vi "Apply VIignore File.vi"(8 "error in":errorcluster, 10 ".VIignore file":path, 11 "VI paths in":path[](array[path])) -> (0 "error out":errorcluster, 2 "Filtered files":string[](array[string]), 3 "VI paths filtered":path[](array[path]))   [LabVIEW 2020, in "CICD.lvlib"]
doc: "Takes in an array of paths and filters them based on filenames in .VIignore file."
uses:
  CICD.lvlib
  65742ef6-5497-4067-8f50-dc0572609d26.vi
  65742ef6-5497-4067-8f50-dc0572609d26.vi/7c7783df-fd5a-49d9-9b7a-63cc9fb0e4e5.vi
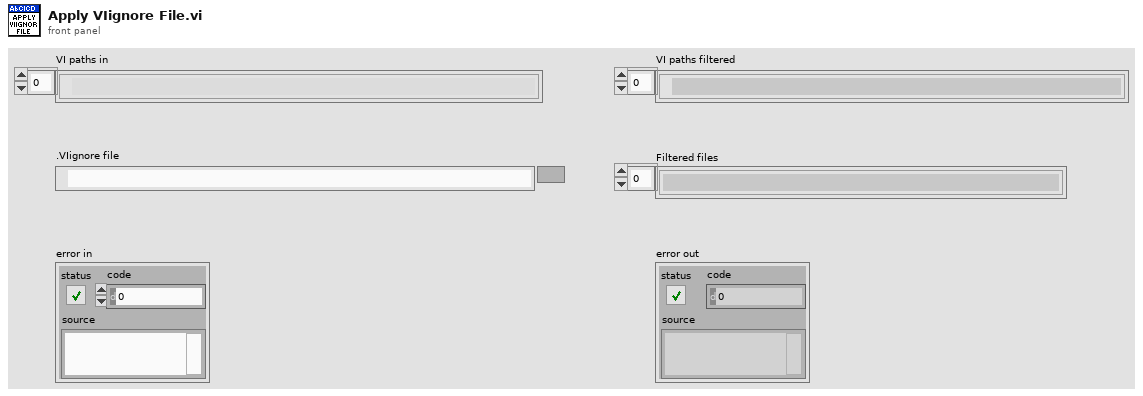
[diagram p1: front panel]
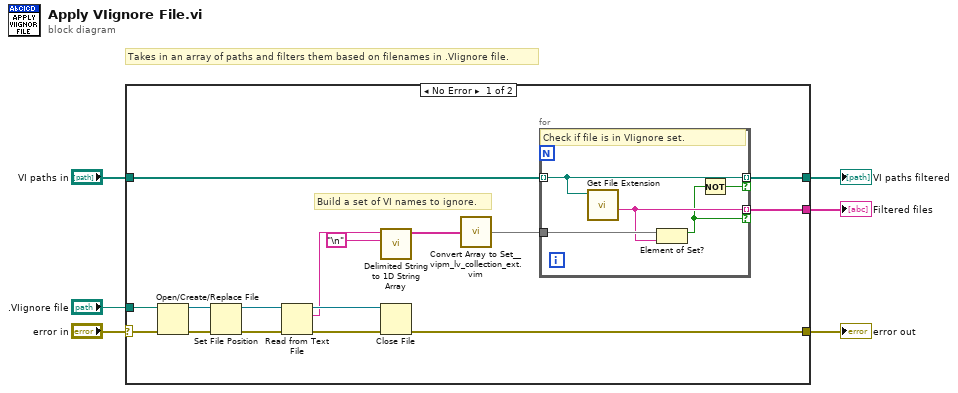
[diagram p0: block diagram]
diagram:
  # "Takes in an array of paths and filters them based on filenames in .VIignore file."
  n1 = case shown="No Error" "error in" {
    selector: "error in" -> [w18 w29]
    tunnel: [w19 w29] -> w6
    tunnel: ".VIignore file" -> [w16 _]
    tunnel: "VI paths in" -> [w11 w28]
    tunnel: [w8 w28] -> w2
    tunnel: [w7 _] -> w1
    frame No Error {
      # "Build a set of VI names to ignore."
      n2 = Open/Create/Replace File(file path (use dialog)=w16, error in=w18) -> (refnum out=w15:refnum<file>, error out=w22:errorcluster)  [unwired: 4 in, 1 out]
      n3 = Set File Position(refnum=w15, error in=w22) -> (refnum out=w14:refnum<file>, error out=w20:errorcluster)  [unwired: 2 in]
      n4 = Read from Text File(file (use dialog)=w14, error in=w20) -> (refnum out=w17:refnum<file>, text=w13:string, error out=w21:errorcluster)  [unwired: 2 in, 1 out]
      n5 = call <vilib>:"Delimited String to 1D String Array.vi"("delimiter"="\n", "delimited string"=w13) -> ("string array"=w10:string[])  [unwired: 9 in]
      n6 = Close File(refnum=w17, error in=w21) -> (error out=w19:errorcluster)  [unwired: 1 out]
      n7 = call "Convert Array to Set__vipm_lv_collection_ext.vim"("array"=w10) -> ("set"=w9:set{string})  [unwired: 6 in]
      n8 = for {
        tunnel: w11 -> [w26] mode=indexing
        tunnel: w9 -> [w27]
        tunnel: [w26] -> w8 mode=indexing if=w24
        tunnel: [w25] -> w7 mode=indexing if=w23
        # "Check if file is in VIignore set."
        n9 = call <vilib>:"Get File Extension.vi"("file"=w26) -> ("filename without extension"=w25:string)  [unwired: 6 in, 4 out]
        n10 = Element of Set?(10:w25, 11:w27) -> (3:w23:bool)
        n11 = Not(x=w23) -> (.not. x?=w24:bool)
      }
    }
    frame Error {
    }
  }
  "VI paths filtered" <- w2
  "error out" <- w6
  "Filtered files" <- w1
